vi "RunEXE.vi"(0 "EXE Path":path, 11 "error in (no error)":errorcluster) -> (4 "Application Ref":refnum<vi>, 15 "error out":errorcluster)   [LabVIEW 2016, in "Drona.lvlib"]
uses:
  Drona.lvlib
  <vilib>/Utility/config.llb/Read Key (I32).vi
  <vilib>/SLL Toolkit/SLL File IO/SLL File IO.lvlib
  <vilib>/Utility/config.llb/NI_LVConfig.lvlib
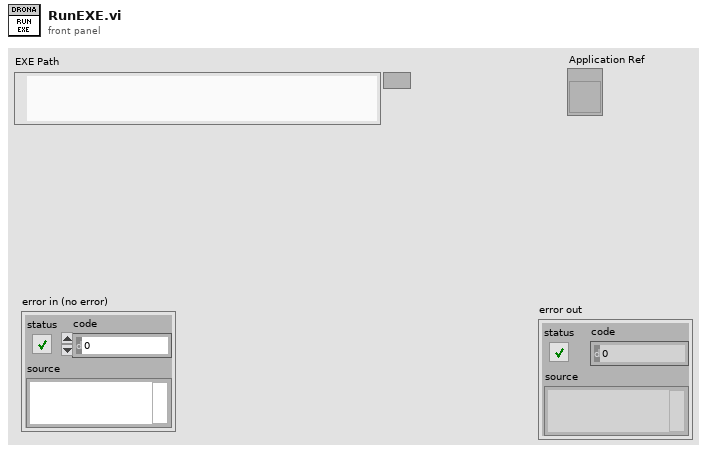
[diagram p1: front panel]
types:
  T1 = typedef "NI_LVConfig.lvlib/Config Data RefNum.ctl" = refnum<k1>
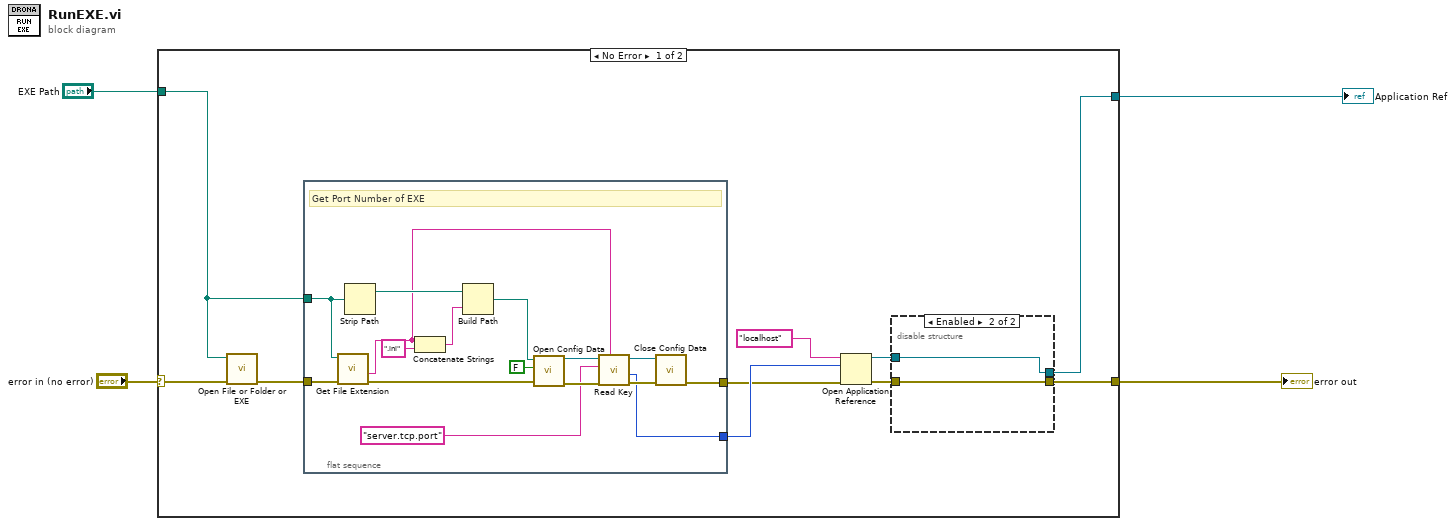
[diagram p0: block diagram]
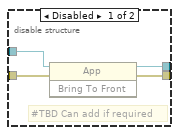
[diagram p2: hidden frame]
diagram:
  n1 = case shown="No Error" "error in (no error)" {
    selector: "error in (no error)" -> [w14 w37]
    tunnel: [w9 w37] -> w3
    tunnel: [w5 _] -> w2
    tunnel: "EXE Path" -> [w12 _]
    frame No Error {
      n2 = call <vilib>:"Open File or Folder or EXE.vi"("error in (no error)"=w14, "Path"=w12) -> ("error out"=w13:errorcluster)  [unwired: 9 in]
      n3 = flat-sequence {
        tunnel: w13 -> [w36]
        tunnel: w12 -> [w35]
        tunnel: [w23] -> w11
        tunnel: [w22] -> w10
        frame #0 {
          # "Get Port Number of EXE"
          n4 = call <vilib>:"Get File Extension.vi"("error in (no error)"=w36, "file"=w35) -> ("error out"=w21:errorcluster, "filename without extension"=w27:string)  [unwired: 5 in, 3 out]
          n5 = Strip Path(path=w35) -> (stripped path=w33:path)  [unwired: 1 out]
          n6 = Concatenate Strings(w27, ".ini" ("string")) -> (w32:string)
          n7 = Build Path(base path=w33, name or relative path=w32) -> (appended path=w31:path)
          n8 = call <vilib>:"Open Config Data.vi"("error in (no error)"=w21, "create file if necessary (T)"=FALSE, "configuration file path"=w31) -> ("error out"=w28:errorcluster, "refnum"=w29:T1)  [unwired: 6 in, 1 out]
          n9 = call-poly <vilib>:"Read Key.vi"("section"=w27, "error in (no error)"=w28, "key"="server.tcp.port", "refnum"=w29) -> ("error out"=w25:errorcluster, "value"=w23:i32, "refnum out"=w24:T1)  [unwired: 4 in, 1 out]
          n10 = call <vilib>:"Close Config Data.vi"("error in (no error)"=w25, "refnum"=w24) -> ("error out"=w22:errorcluster)  [unwired: 8 in, 1 out]
        }
      }
      n11 = Open Application Reference(8:w10, 10:w11, 11:"localhost" ("machine name (\"\":  open local reference)")) -> (0:w7:errorcluster, 3:w6:refnum<vi>)  [unwired: 1 in]
      n12 = disable-structure shown="Enabled" {
        disable-tunnel: [w18 w20] -> w9
        disable-tunnel: w7 -> [w17 w20]
        disable-tunnel: w6 -> [w16 w19]
        disable-tunnel: [w15 w19] -> w5
        frame Disabled {
          # "#TBD Can add if required"
          n13 = invoke class="App" method="Bring To Front"(reference=w16, error in=w17) -> (reference out=w15:refnum<vi>, error out=w18:errorcluster)  [unwired: 1 in, 1 out]
        }
        frame Enabled {
        }
      }
    }
    frame Error {
    }
  }
  "error out" <- w3
  "Application Ref" <- w2
